vi "UI Producer Consumer 2012 NIVerified.vi"() -> ()   [LabVIEW 2020]
doc: "This VI illustrates an architecture that allows the user to queue multiple processes. Each process contains multiple state, or in this case stages.The queueing of events is handled by the producer UI loop while the consumer loop goes through each process' states. The processes can have functionality different from one another or can have the same functionality. This architecture allows for expansion on the number of processes as well as the number of states for each process by augmenting the states enum and inputting state functionality in the state case. I have changed the consumer loop to have a time of 500 ms in order to make it easier for the user to enqueue elements. The slowed down consumer loops allowed queue processes to build due to the slow progression of the queue. To hasten the program, the user can change the time constant.\n\nThis type of architecture can apply to an application containing multiple processes, who each have multiple states. This allows the user to easily queue up processes that will proceed in the order that the user selects. There is also two different stop functionalities in order to ensure that a current process is completed or that the current state is completed before stopping the program. This can easily be scaled by editing the type-def enum and adding states to the state machine."
uses:
  States.ctl
panel:
  in  "Emergency Stop Button":bool
  out "Queue":T1[](array[typedef])
  out "Cluster":T2
  in  "Stop Button":bool
  in  "Process 3":bool
  in  "Process 2":bool
  in  "Process 1":bool
  # "Overview: A producer/consumer architecture with a UI producer loop and a state machine consumer loop. Allows the user to queue multiple state sequences.\nRequirements: LabVIEW 2012 (or compatible\nInstructions:\n1. Run the VI.\n2. Press various Process buttons to see the Queue build.\n3. See the Process and Stage in the Cluster of Boolean indicators.\n4. Press Stop during Process to see Stop functionality.\n5. Run VI again after the program has stopped.\n6. Repeat step 2.\n7. Press Emergency Stop button to see Emergency Stop functionality."
  # "Click the Process button of your choice to enqueue the process of your choice. \nThe Processes will execute in the order that you queue them in."
  # "Stop Button stops program after current process has finished"
  # "Emergency Stop Button stops program after the current state. Press this button to stop in the middle of a Process"
  # "Shows the current Queue."
  # "The Boolean Cluster shows you what process is occurring and the stage it is on.\nEach stage corresponds to a state in a process."
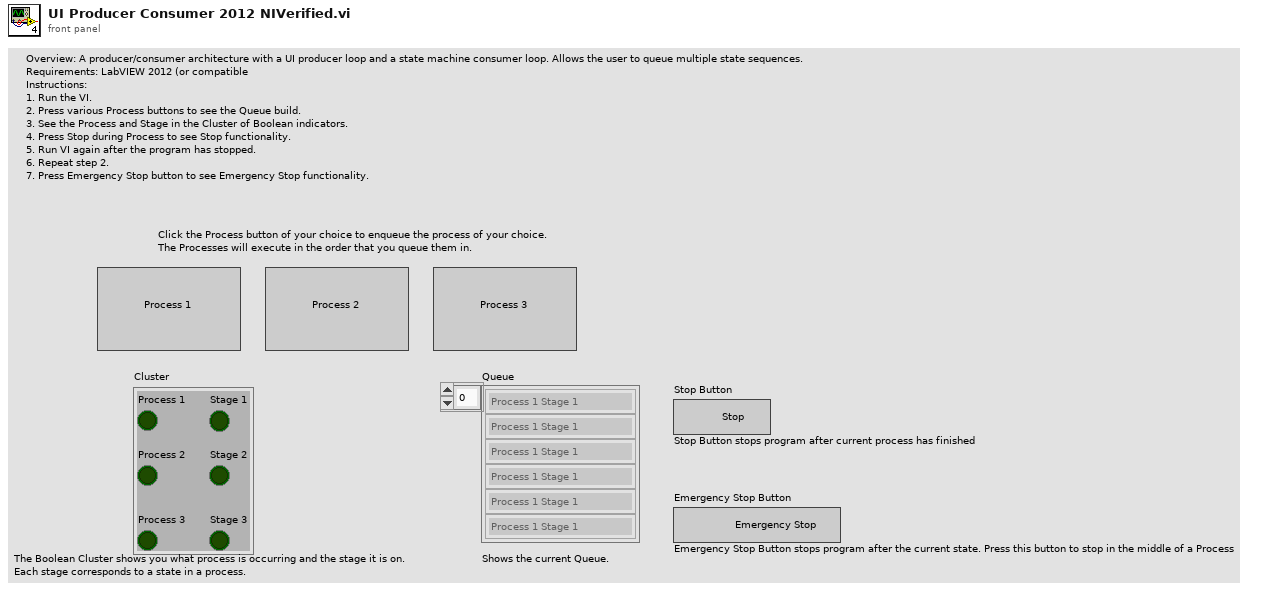
[diagram p1: front panel]
types:
  T1 = typedef "States.ctl" = enum16{"Process 1 Stage 1", "Process 1 Stage 2", "Process 1 Stage 3", "Process 2 Stage 1", "Process 2 Stage 2", "Process 2 Stage 3", "Process 3 Stage 1", "Process 3 Stage 2", "Process 3 Stage 3", "Wait", "Stop", "Emergency Stop"}
  T2 = cluster{"Process 1":bool, "Stage 1":bool, "Process 2":bool, "Stage 2":bool, "Process 3":bool, "Stage 3":bool}
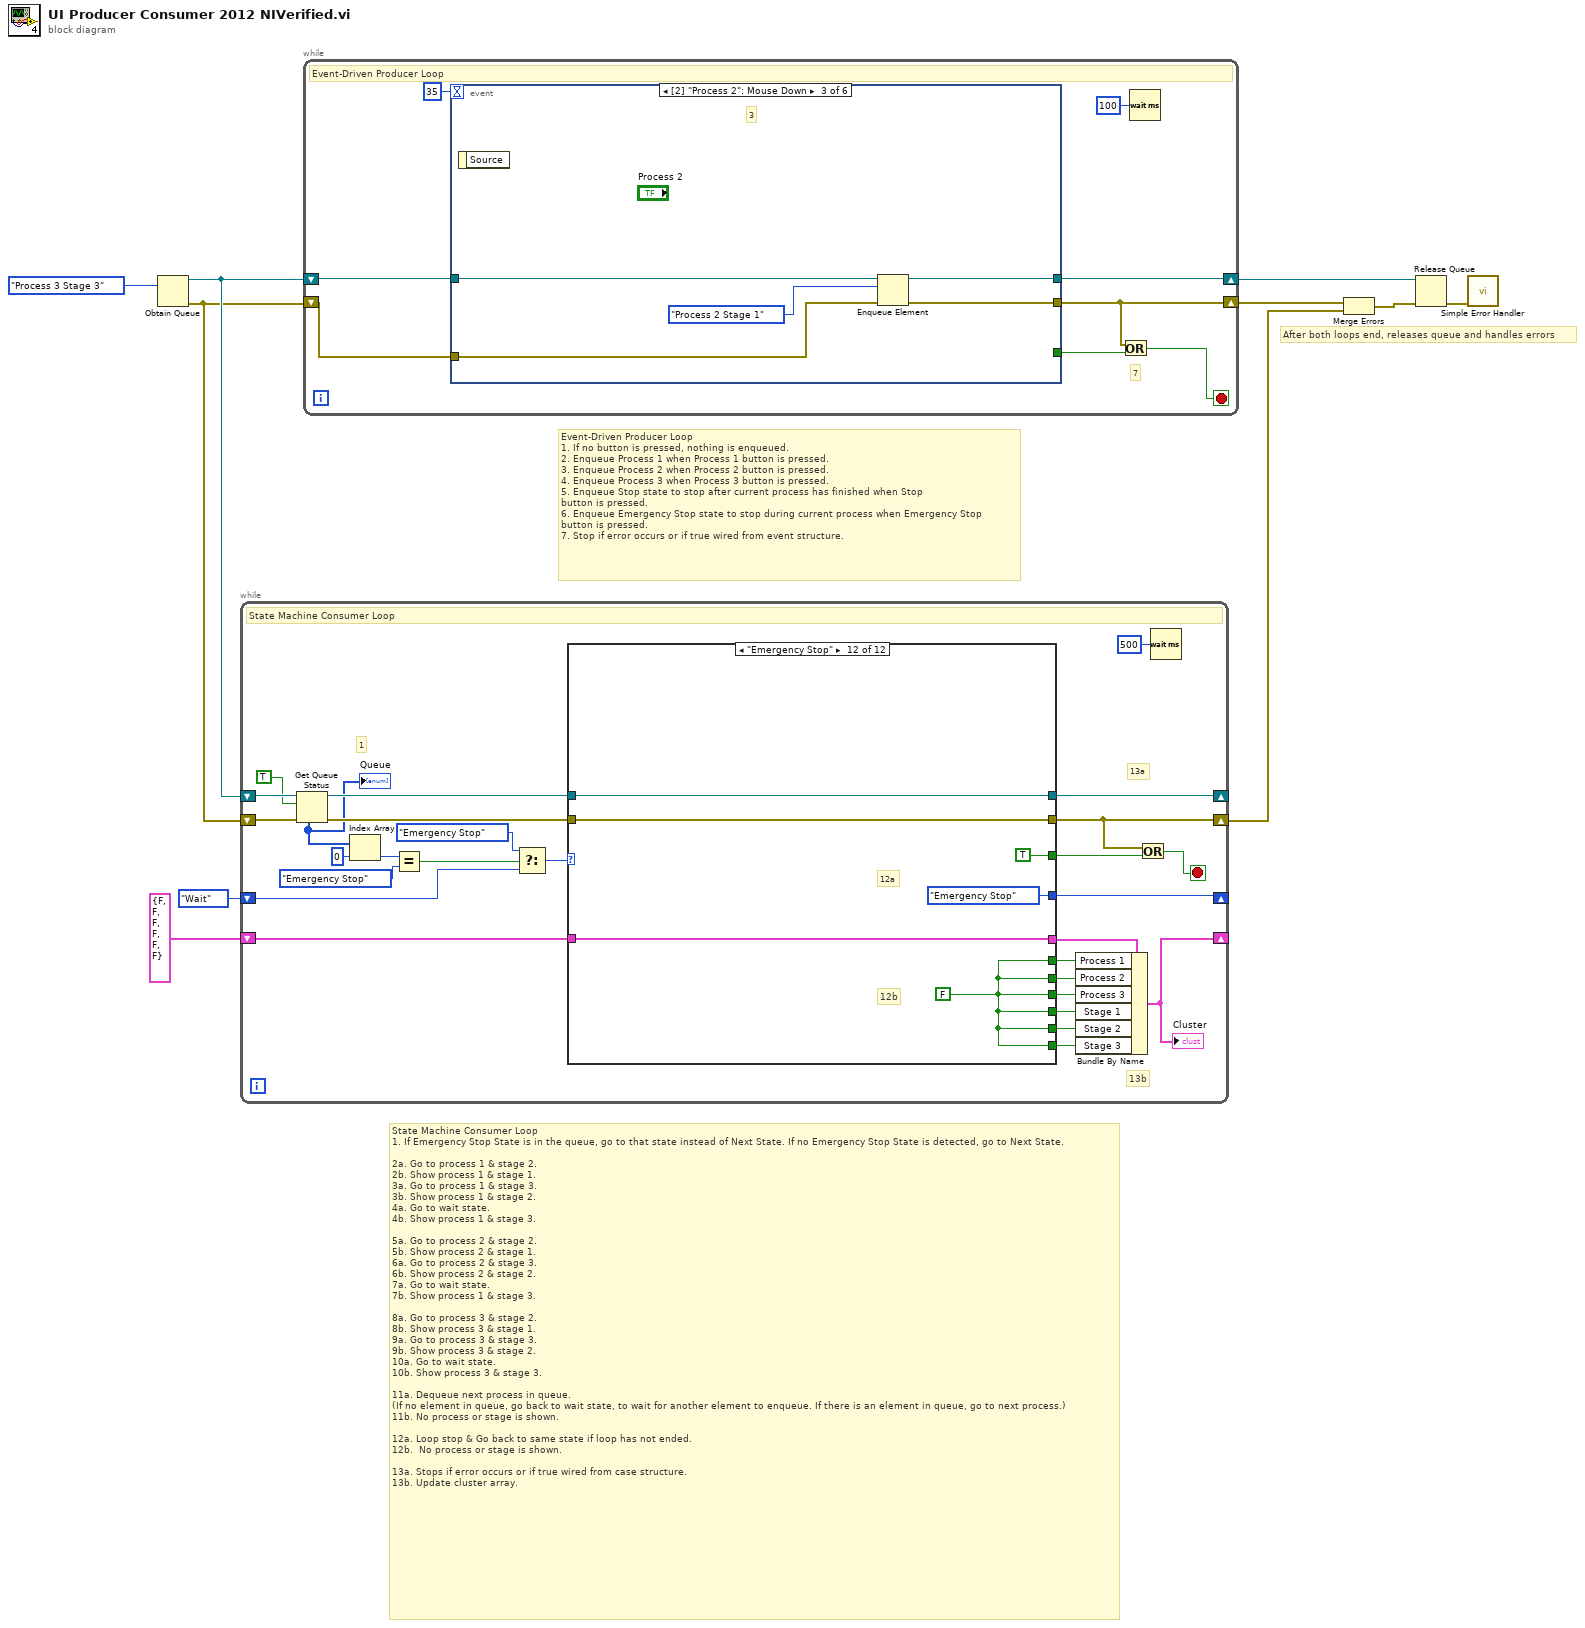
[diagram p0: block diagram]
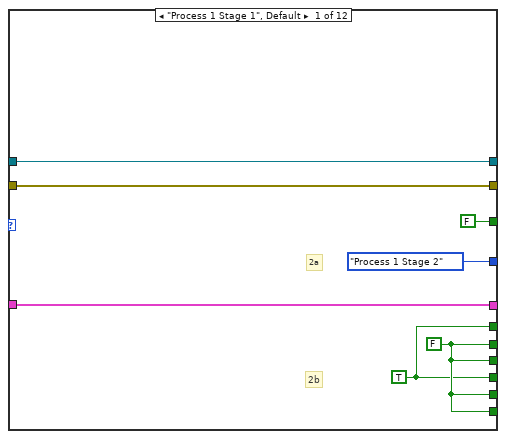
[diagram p2: hidden frame]
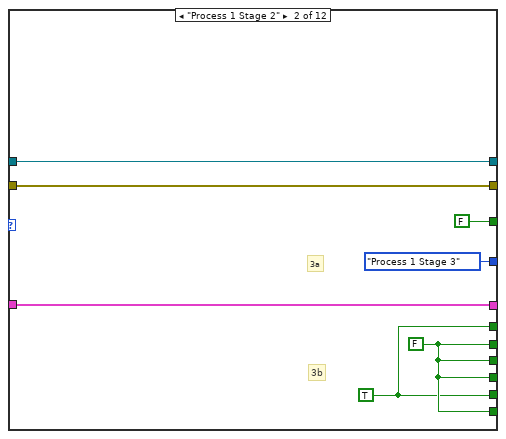
[diagram p3: hidden frame]
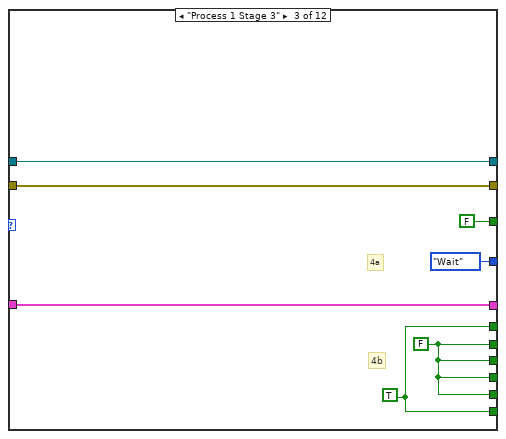
[diagram p4: hidden frame]
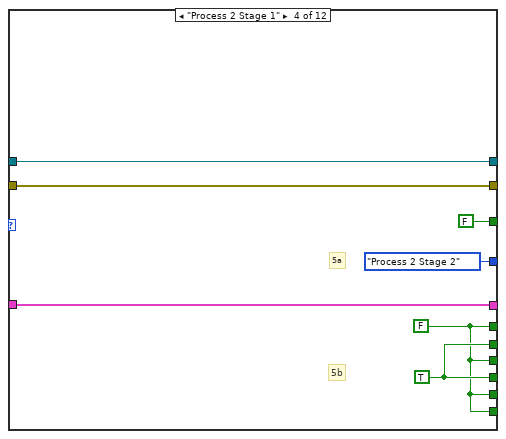
[diagram p5: hidden frame]
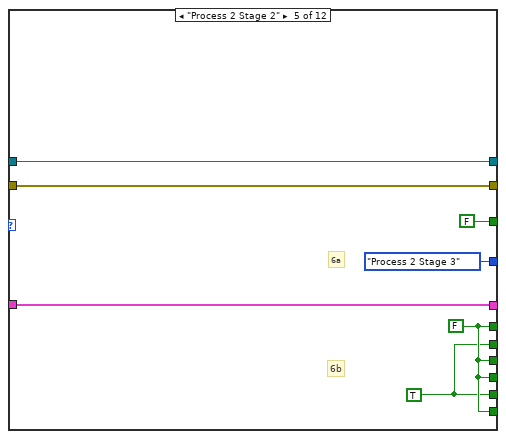
[diagram p6: hidden frame]
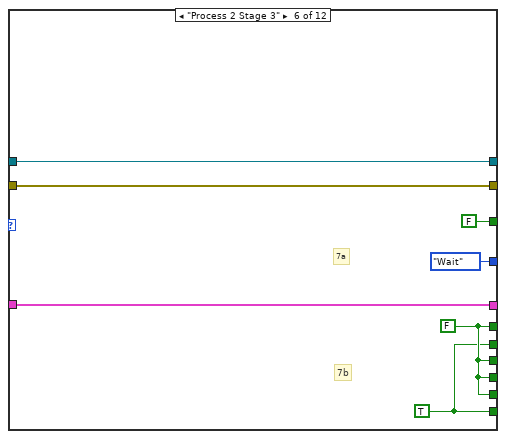
[diagram p7: hidden frame]
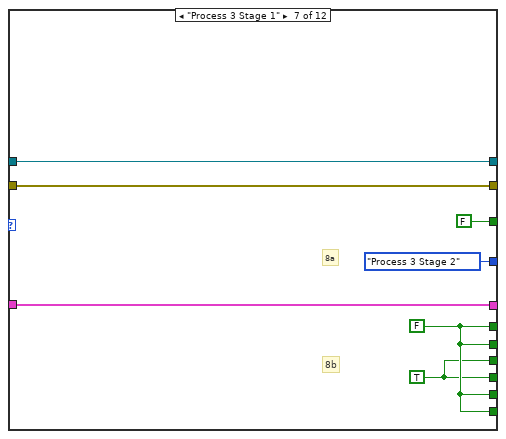
[diagram p8: hidden frame]
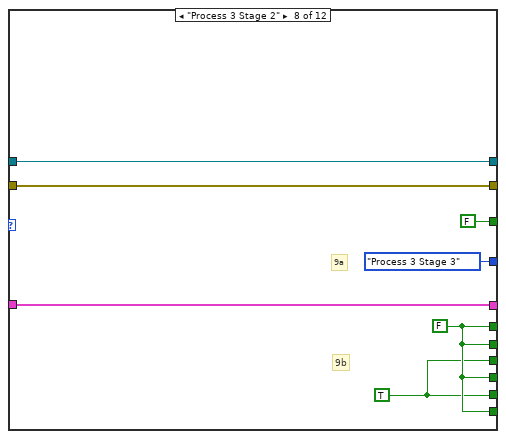
[diagram p9: hidden frame]
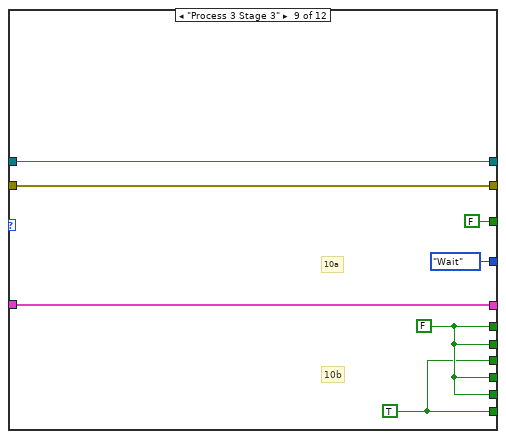
[diagram p10: hidden frame]
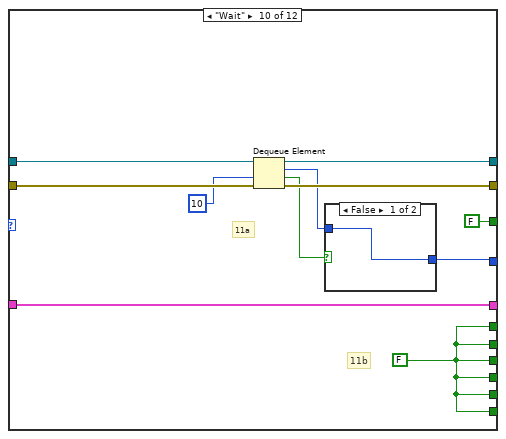
[diagram p11: hidden frame]
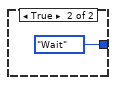
[diagram p12: hidden frame]
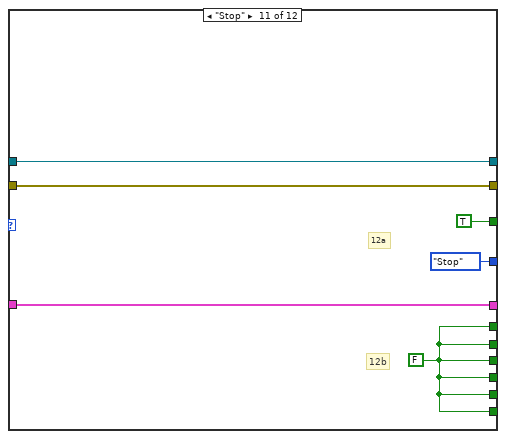
[diagram p13: hidden frame]
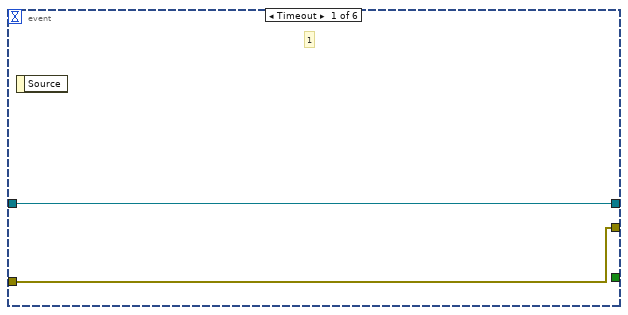
[diagram p14: hidden frame]
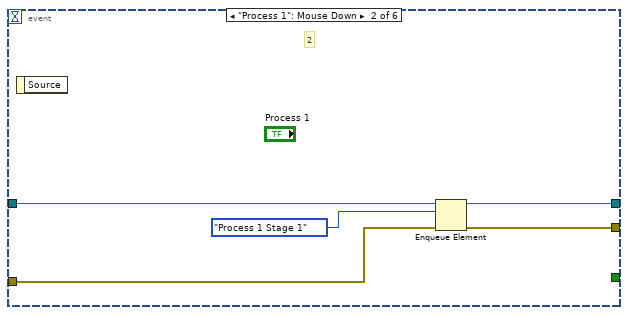
[diagram p15: hidden frame]
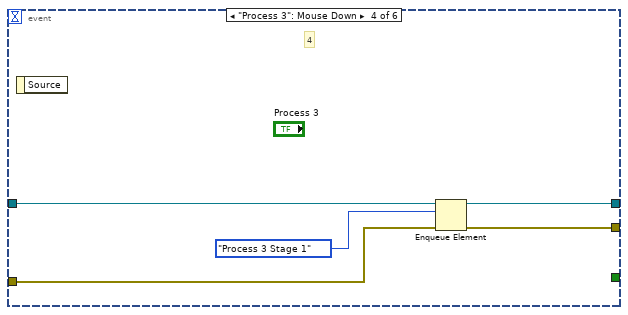
[diagram p16: hidden frame]
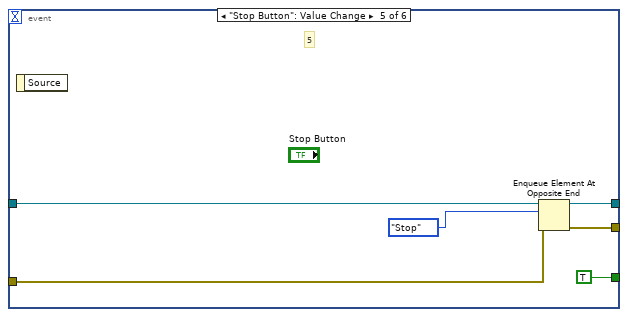
[diagram p17: hidden frame]
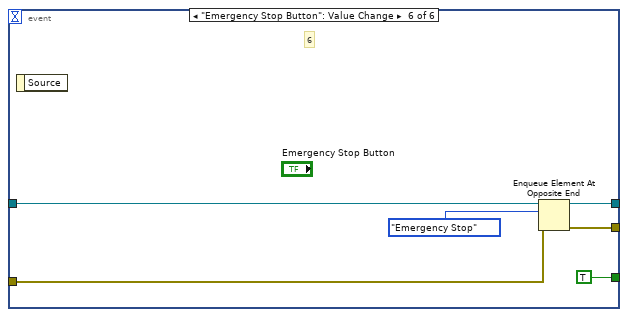
[diagram p18: hidden frame]
diagram:
  # "State Machine Consumer Loop\n1. If Emergency Stop State is in the queue, go to that state instead of Next State. If no Emergency Stop State is detected, go to Next State.\n\n2a. Go to process 1 & stage 2.\n2b. Show process 1 & stage 1.\n3a. Go to process 1 & stage 3.\n3b. Show process 1 & stage 2.\n4a. Go to wait state.\n4b. Show process 1 & stage 3.\n\n5a. Go to process 2 & stage 2.\n5b. Show process 2 & stage 1.\n6a. Go to process 2 & stage 3.\n6b. Show process 2 & stage 2.\n7a. Go to wait state.\n7b. Show process 1 & stage 3.\n\n8a. Go to process 3 & stage 2.\n8b. Show process 3 & stage 1.\n9a. Go to process 3 & stage 3.\n9b. Show process 3 & stage 2.\n10a. Go to wait state.\n10b. Show process 3 & stage 3.\n\n11a. Dequeue next process in queue.\n(If no element in queue, go back to wait state, to wait for another element to enqueue. If there is an element in queue, go to next process.)\n11b. No process or stage is shown.\n\n12a. Loop stop & Go back to same state if loop has not ended.\n12b.  No process or stage is shown.\n\n13a. Stops if error occurs or if true wired from case structure.\n13b. Update cluster array."
  # "Event-Driven Producer Loop\n1. If no button is pressed, nothing is enqueued.\n2. Enqueue Process 1 when Process 1 button is pressed.\n3. Enqueue Process 2 when Process 2 button is pressed.\n4. Enqueue Process 3 when Process 3 button is pressed.\n5. Enqueue Stop state to stop after current process has finished when Stop\nbutton is pressed.\n6. Enqueue Emergency Stop state to stop during current process when Emergency Stop\nbutton is pressed.\n7. Stop if error occurs or if true wired from event structure."
  # "After both loops end, releases queue and handles errors"
  n1 = Obtain Queue(element data type=States."Process 3 Stage 3") -> (queue out=w10:refnum<queue>, error out=w9:errorcluster)  [unwired: 4 in, 1 out]
  n2 = while {
    shift-right: [w24] -> _
    shift-left: w10 -> [w36]
    shift-right: [w20] -> w1
    shift-left: w9 -> [w35]
    shift-right: [w23] -> _
    shift-left: States."Wait" ("y") -> [w13]
    shift-right: [w31] -> _
    shift-left: T2 {"Process 1"=FALSE, "Stage 1"=FALSE, "Process 2"=FALSE, "Stage 2"=FALSE, "Process 3"=FALSE, "Stage 3"=FALSE} ("Cluster") -> [w33]
    stop <- w38 stop-if-true
    # "13a"
    # "13b"
    # "1"
    # "State Machine Consumer Loop"
    n3 = Get Queue Status(queue=w36, return elements? (F)=TRUE, error in (no error)=w35) -> (queue out=w34:refnum<queue>, error out=w21:errorcluster, elements=w18:T1[])  [unwired: 5 out]
    "Queue" <- w18
    n4 = Index Array(array=w18, index=0) -> (element=w16:T1)
    n5 = Equal?(x=w16, y=States."Emergency Stop") -> (x = y?=w14:bool)
    n6 = Select(t=States."Emergency Stop", s=w14, f=w13) -> (s? t:f=w11:T1)
    n7 = case shown="\"Emergency Stop\"" w11 {
      tunnel: w34 -> [w42 w49 w58 w65 w72 w79 w86 w93 w100 w110 w120 w126]
      tunnel: w21 -> [w41 w48 w57 w64 w71 w78 w85 w92 w99 w109 w119 w125]
      tunnel: w33 -> [w45 w52 w59 w66 w73 w80 w87 w94 w101 w112 w118 w124]
      tunnel: [w45 w52 w59 w66 w73 w80 w87 w94 w101 w112 w118 w124] -> w32
      tunnel: [w43 w50 w55 w62 w70 w77 w84 w91 w98 w111 w117 w123] -> w30
      tunnel: [w44 w50 w56 w62 w69 w77 w84 w90 w98 w111 w117 w123] -> w29
      tunnel: [w44 w51 w56 w63 w69 w76 w84 w91 w98 w111 w117 w123] -> w28
      tunnel: [w44 w51 w56 w62 w70 w77 w83 w90 w97 w111 w117 w123] -> w27
      tunnel: [w43 w51 w56 w63 w70 w77 w83 w91 w98 w111 w117 w123] -> w26
      tunnel: [w44 w51 w55 w62 w70 w76 w84 w91 w97 w111 w117 w123] -> w25
      tunnel: [w42 w49 w58 w65 w72 w79 w86 w93 w100 w108 w120 w126] -> w24
      tunnel: [w41 w48 w57 w64 w71 w78 w85 w92 w99 w107 w119 w125] -> w20
      tunnel: [States."Process 1 Stage 2" ("y") States."Process 1 Stage 3" ("y") States."Wait" ("y") States."Process 2 Stage 2" ("y") States."Process 2 Stage 3" ("y") States."Wait" ("y") States."Process 3 Stage 2" ("y") States."Process 3 Stage 3" ("y") States."Wait" ("y") w104 States."Stop" ("y") States."Emergency Stop" ("y")] -> w23
      tunnel: [FALSE FALSE FALSE FALSE FALSE FALSE FALSE FALSE FALSE FALSE TRUE TRUE] -> w22
      frame "Process 1 Stage 1", Default {
        w43 = TRUE
        w44 = FALSE
        # "2b"
        # "2a"
      }
      frame "Process 1 Stage 2" {
        w51 = FALSE
        w50 = TRUE
        # "3b"
        # "3a"
      }
      frame "Process 1 Stage 3" {
        w56 = FALSE
        w55 = TRUE
        # "4b"
        # "4a"
      }
      frame "Process 2 Stage 1" {
        w62 = FALSE
        w63 = TRUE
        # "5b"
        # "5a"
      }
      frame "Process 2 Stage 2" {
        w70 = FALSE
        w69 = TRUE
        # "6a"
        # "6b"
      }
      frame "Process 2 Stage 3" {
        w77 = FALSE
        w76 = TRUE
        # "7a"
        # "7b"
      }
      frame "Process 3 Stage 1" {
        w84 = FALSE
        w83 = TRUE
        # "8b"
        # "8a"
      }
      frame "Process 3 Stage 2" {
        w91 = FALSE
        w90 = TRUE
        # "9a"
        # "9b"
      }
      frame "Process 3 Stage 3" {
        w98 = FALSE
        w97 = TRUE
        # "10a"
        # "10b"
      }
      frame "Wait" {
        w111 = FALSE
        # "11b"
        # "11a"
        n8 = Dequeue Element(queue=w110, timeout in ms (-1)=10, error in (no error)=w109) -> (queue out=w108:refnum<queue>, element=w105:T1, timed out?=w106:bool, error out=w107:errorcluster)
        n9 = case shown="False" w106 {
          tunnel: w105 -> [w113 _]
          tunnel: [w113 States."Wait" ("y")] -> w104
          frame False {
          }
          frame True {
          }
        }
      }
      frame "Stop" {
        w117 = FALSE
        # "12a"
        # "12b"
      }
      frame "Emergency Stop" {
        w123 = FALSE
        # "12b"
        # "12a"
      }
    }
    n10 = Bundle By Name(cluster=w32, "Process 1"=w30, "Process 2"=w28, "Process 3"=w27, "Stage 1"=w26, "Stage 2"=w29, "Stage 3"=w25) -> (w31:T2)
    "Cluster" <- w31
    n11 = Or(x=w20, y=w22) -> (x .or. y?=w38:bool)
    n12 = Wait (ms)(milliseconds to wait=u32 500) -> ()  [unwired: 1 out]
  }
  n13 = while {
    shift-right: [w131] -> w6
    shift-left: w10 -> [w133]
    shift-right: [w130] -> w8
    shift-left: w9 -> [w132]
    stop <- w128 stop-if-true
    # "7"
    # "Event-Driven Producer Loop"
    n14 = event shown="[2] \"Process 2\": Mouse Down" {
      selector: _ -> [_ _ _ _ _ _]
      dyn-events: _ -> [_ _ _ _ _ _]
      timeout: 35 -> [_ _ _ _ _ _]
      tunnel: w133 -> [w136 w141 w146 w151 w157 w163]
      tunnel: w132 -> [w135 w139 w144 w149 w156 w162]
      tunnel: [w135 w138 w143 w148 w154 w160] -> w130
      tunnel: [w136 w140 w145 w150 w155 w161] -> w131
      tunnel: [_ _ _ _ TRUE TRUE] -> w129
      event Timeout {
        # "1"
        n15 = event-data() -> ()  [unwired: 1 in, 1 out]
      }
      event "Process 1": Mouse Down {
        # "2"
        n16 = event-data() -> ()  [unwired: 1 in, 1 out]
        n17 = Enqueue Element(queue=w141, element=States."Process 1 Stage 1", error in (no error)=w139) -> (queue out=w140:refnum<queue>, error out=w138:errorcluster)  [unwired: 1 in, 1 out]
      }
      event "Process 2": Mouse Down {
        # "3"
        n18 = event-data() -> ()  [unwired: 1 in, 1 out]
        n19 = Enqueue Element(queue=w146, element=States."Process 2 Stage 1", error in (no error)=w144) -> (queue out=w145:refnum<queue>, error out=w143:errorcluster)  [unwired: 1 in, 1 out]
      }
      event "Process 3": Mouse Down {
        # "4"
        n20 = event-data() -> ()  [unwired: 1 in, 1 out]
        n21 = Enqueue Element(queue=w151, element=States."Process 3 Stage 1", error in (no error)=w149) -> (queue out=w150:refnum<queue>, error out=w148:errorcluster)  [unwired: 1 in, 1 out]
      }
      event "Stop Button": Value Change {
        # "5"
        n22 = event-data() -> ()  [unwired: 1 in, 1 out]
        n23 = Enqueue Element At Opposite End(queue=w157, element=States."Stop", error in (no error)=w156) -> (queue out=w155:refnum<queue>, error out=w154:errorcluster)  [unwired: 1 in, 1 out]
      }
      event "Emergency Stop Button": Value Change {
        # "6"
        n24 = event-data() -> ()  [unwired: 1 in, 1 out]
        n25 = Enqueue Element At Opposite End(queue=w163, element=States."Emergency Stop", error in (no error)=w162) -> (queue out=w161:refnum<queue>, error out=w160:errorcluster)  [unwired: 1 in, 1 out]
      }
    }
    n26 = Or(x=w130, y=w129) -> (x .or. y?=w128:bool)
    n27 = Wait (ms)(milliseconds to wait=u32 100) -> ()  [unwired: 1 out]
  }
  n28 = Merge Errors(w8, w1) -> (w7:errorcluster)
  n29 = Release Queue(queue=w6, error in (no error)=w7) -> (error out=w3:errorcluster)  [unwired: 1 in, 2 out]
  n30 = call <vilib>:"Simple Error Handler.vi"("error in (no error)"=w3) -> ()  [unwired: 4 in, 5 out]
